vi "Init.vi"(8 "error in (no error)":errorcluster, 11 "Submissions":path) -> (0 "error out":errorcluster, 3 "Submit out":refnum<class "Submit.lvclass">)   [LabVIEW 2020, in "Summer of LabVIEW.lvlib" / "Submit.lvclass"]
uses:
  Submit.lvclass
  Submit.lvclass/Submit.ctl
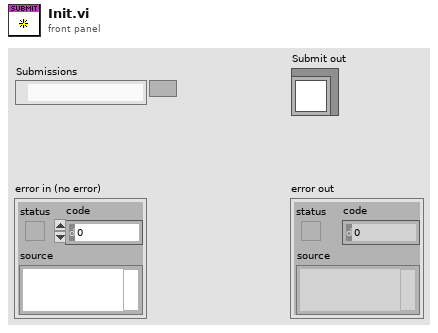
[diagram p1: front panel]
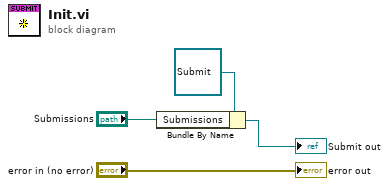
[diagram p0: block diagram]
diagram:
  n1 = Bundle By Name(cluster=refnum<class "Submit.lvclass"> refnum ("Submit in"), "Submissions"="Submissions") -> (→"Submit out":refnum<class "Submit.lvclass">)
  "error out" <- "error in (no error)"
